vi "Check Run Build.vi"(8 "error in (no error)":errorcluster, 10 "Run":refnum<class>, 11 "Kasli in":refnum<class "Kasli.lvclass">) -> (0 "error out":errorcluster, 2 "Correct Build":bool)   [LabVIEW 2020, in "Kasli Wrapper 2.0.lvlib" / "Kasli.lvclass"]
uses:
  Kasli.lvclass
  Run Utilities/Run Instance/Run Instance.lvclass
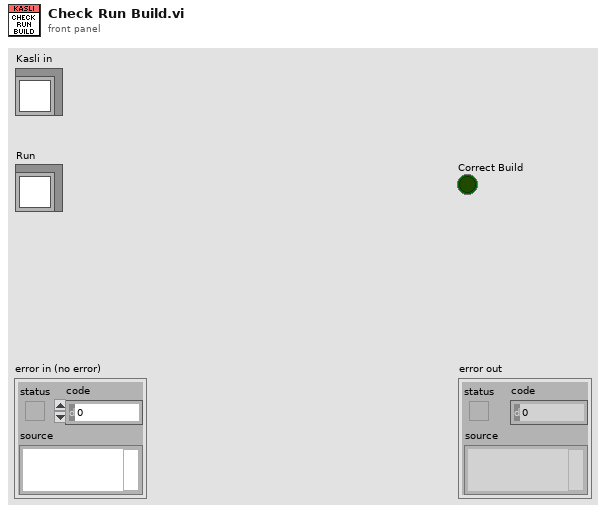
[diagram p1: front panel]
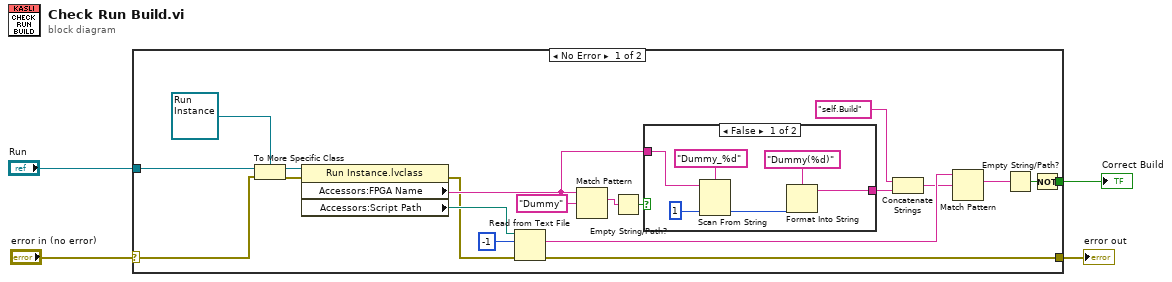
[diagram p0: block diagram]
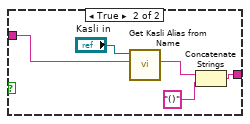
[diagram p2: hidden frame]
diagram:
  n1 = case shown="No Error" "error in (no error)" {
    selector: "error in (no error)" -> [w6 w36]
    tunnel: [w18 w36] -> w3
    tunnel: "Run" -> [w20 _]
    tunnel: [w17 _] -> w1
    frame No Error {
      n2 = To More Specific Class(target class=refnum<class "Run Instance.lvclass"> refnum ("Run"), reference=w20, error in=w6) -> (specific class reference=w9:refnum<class "Run Instance.lvclass">, error out=w7:errorcluster)
      n3 = property class="Run Instance.lvclass"(reference=w9, error in=w7) -> (error out=w5:errorcluster, "Accessors:FPGA Name"=w10:string, "Accessors:Script Path"=w19:path)  [unwired: 1 out]
      n4 = Read from Text File(file (use dialog)=w19, count=-1, error in=w5) -> (text=w23:string, error out=w18:errorcluster)  [unwired: 1 in, 2 out]
      n5 = Match Pattern(string=w10, regular expression="Dummy") -> (match substring=w14:string)  [unwired: 1 in, 3 out]
      n6 = Empty String/Path?(string/path=w14) -> (empty?=w15:bool)
      n7 = case shown="False" w15 {
        tunnel: [w25 w35] -> w13
        tunnel: w10 -> [w30 w31]
        frame False {
          n8 = Scan From String(format string="Dummy_%d", input string=w30, default 1=1) -> (output 1=w27:i32)  [unwired: 2 in, 3 out]
          n9 = Format Into String(format string="Dummy(%d)", w27) -> (resulting string=w25:string)  [unwired: 2 in, 1 out]
        }
        frame True {
          n10 = call-dynamic "Get Kasli Alias from Name.vi"("Kasli Name"=w31, "Kasli in"="Kasli in") -> ("Kasli Alias"=w32:string)  [unwired: 7 in, 2 out]
          n11 = Concatenate Strings(w32, "()" ("string")) -> (w35:string)
        }
      }
      n12 = Concatenate Strings("self.Build" ("regular expression"), w13) -> (w11:string)
      n13 = Match Pattern(string=w23, regular expression=w11) -> (match substring=w22:string)  [unwired: 1 in, 3 out]
      n14 = Empty String/Path?(string/path=w22) -> (empty?=w21:bool)
      n15 = Not(x=w21) -> (.not. x?=w17:bool)
    }
    frame Error {
    }
  }
  "error out" <- w3
  "Correct Build" <- w1
